vi "Impose Velocity Limits.vi"(9 "Array":dbl[](array[numeric]), 10 "Values in":cluster{"accel":dbl, "velocity":dbl}, 11 "Ends":cluster{"Accel End":bool, "Decel End":bool}) -> (2 "Values out":cluster{"accel":dbl, "velocity":dbl})   [LabVIEW 2025]
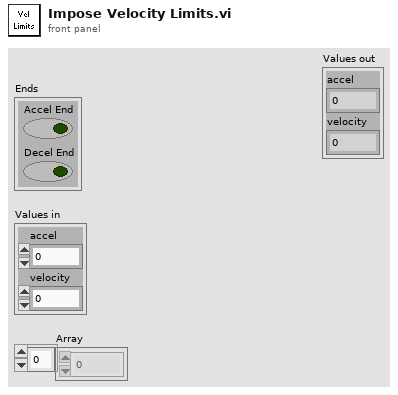
[diagram p1: front panel]
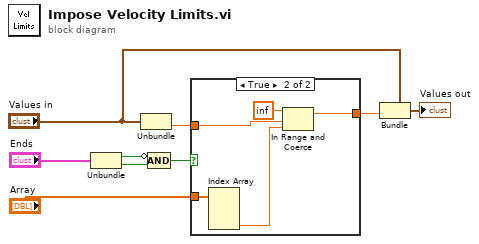
[diagram p0: block diagram]
diagram:
  n1 = Unbundle("Ends") -> ("Accel End"=w8:bool, "Decel End"=w7:bool)
  n2 = Unbundle("Values in") -> ("velocity"=w4:dbl)  [unwired: 1 out]
  n3 = Compound Arithmetic op=AND(invert w8, w7) -> (w6:bool)
  n4 = case shown="True" w6 {
    tunnel: "Array" -> [_ w15]
    tunnel: [w10 w12] -> w3
    tunnel: w4 -> [w10 w11]
    frame False {
    }
    frame True {
      n5 = Index Array(array=w15) -> (element #3=w14:dbl)  [unwired: 3 in, 2 out]
      n6 = In Range and Coerce(upper limit=inf, x=w11, lower limit=w14) -> (coerced(x)=w12:dbl)  [unwired: 1 out]
    }
  }
  n7 = Bundle(cluster="Values in", "velocity"=w3) -> (→"Values out":cluster{"accel":dbl, "velocity":dbl})  [unwired: 1 in]
